vi "Day1_SineWave.vi"() -> ()   [LabVIEW 2025]
panel:
  in  "Knob":dbl(knob) scale=0.0..10.0
  in  "stop":bool
  out "Waveform Chart":dynamicdata(graph)
  # "Knob - The frequency values in Hz; so when the knob points to 2, the sine wave cycles at 2Hz (2 waves per second)"
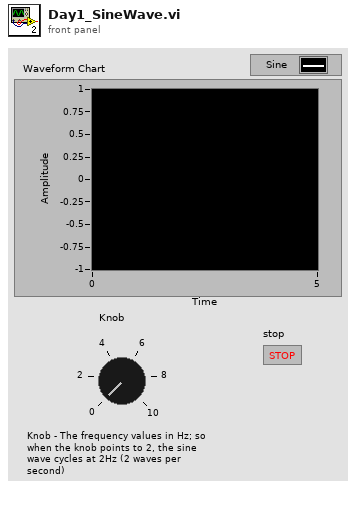
[diagram p1: front panel]
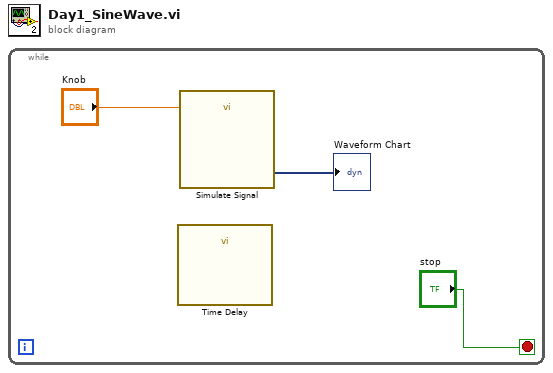
[diagram p0: block diagram]
diagram:
  n1 = while {
    stop <- "stop" stop-if-true
    n2 = call "Time Delay"() -> ()  [unwired: 11 in, 1 out]
    n3 = call "Simulate Signal"("Frequency"="Knob") -> ("Sine"=→"Waveform Chart":dynamicdata)  [unwired: 13 in, 1 out]
  }
